vi "Place in Variant.vi"(9 "error in (no error)":errorcluster, 10 "object":refnum<class "JSON Value.lvclass">, 11 "wire type":refnum<class "JSON Value.lvclass">) -> (1 "error out":errorcluster, 2 "variant (of wire type, containing object)":variant)   [LabVIEW 2011, in "JSON Value.lvclass"]
doc: "Places the supplied JSON Value object in a Variant that has the wire type of the type input. The wire type must be set correctly so that \"Variant to Data\" will accept it without error. Any subclass of JSON Value must override this method with a copy that just changes the class of the type input."
uses:
  JSON Value.lvclass
panel:
  # "wire type"
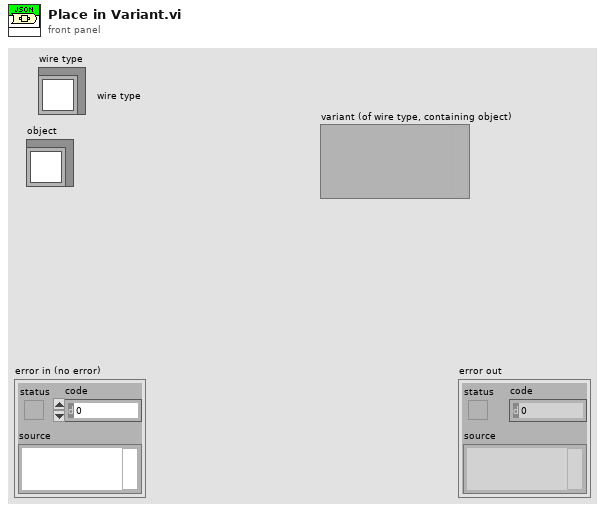
[diagram p1: front panel]
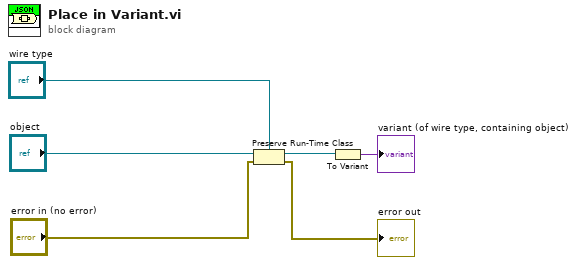
[diagram p0: block diagram]
diagram:
  n1 = Preserve Run-Time Class(object in="object", error in="error in (no error)", 2:"wire type") -> (object out=w2:refnum<class "JSON Value.lvclass">, error out=→"error out":errorcluster)
  n2 = To Variant(anything=w2) -> (Variant=→"variant (of wire type, containing object)":variant)
